vi "Bring To Cursor.vi"(8 "error in (no error)":errorcluster, 11 "Palette Data":T1) -> (0 "error out":errorcluster)   [LabVIEW 2014, in "SmartPalette.lvlib"]
uses:
  SmartPalette.lvlib
  Controls/Palette Data.ctl
  <vilib>/picture/picture.llb/imagedata.ctl
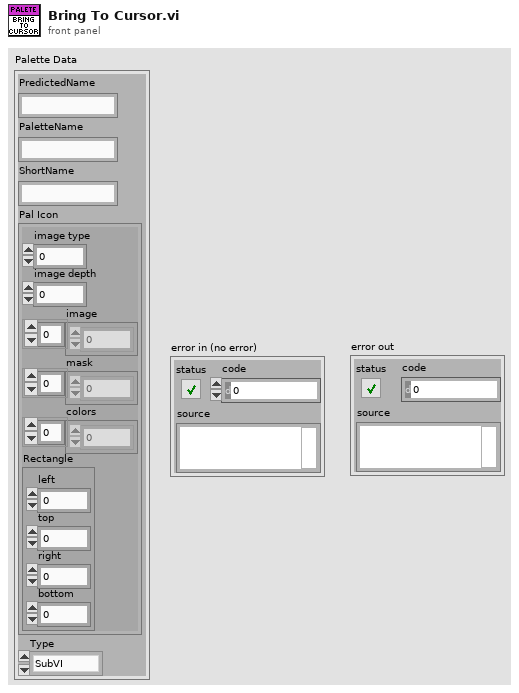
[diagram p1: front panel]
types:
  T1 = typedef "SmartPalette.lvlib/Palette Data.ctl" = cluster{"PredictedName":string, "PaletteName":string, "ShortName":string, "Pal Icon":T2, "Type":enum16{"SubVI", "VI Templtate", "Function"}}
  T2 = typedef "imagedata.ctl" = cluster{"image type":i32, "image depth":i32, "image":u8[], "mask":u8[], "colors":u32[], "Rectangle":cluster{"left":i16, "top":i16, "right":i16, "bottom":i16}}
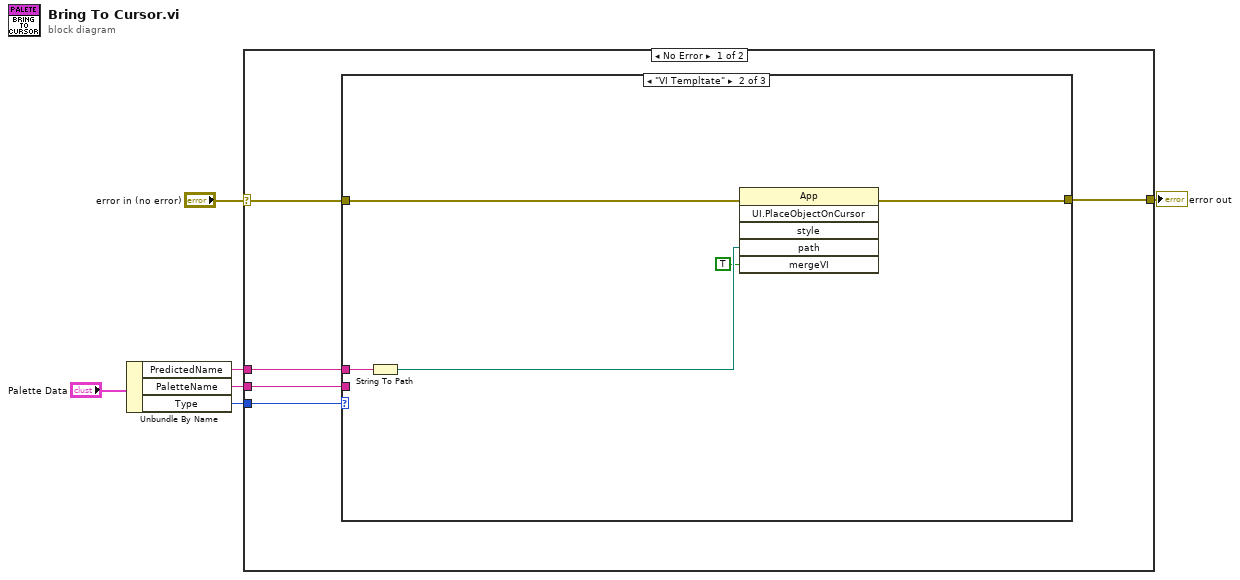
[diagram p0: block diagram]
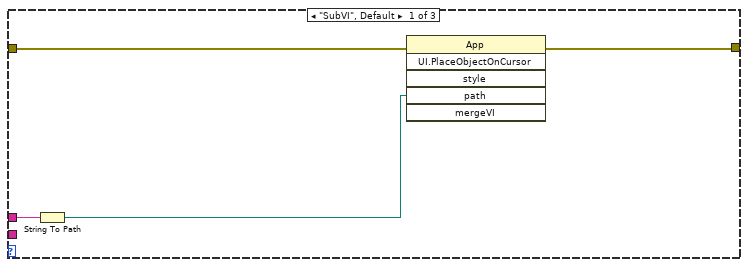
[diagram p2: hidden frame]
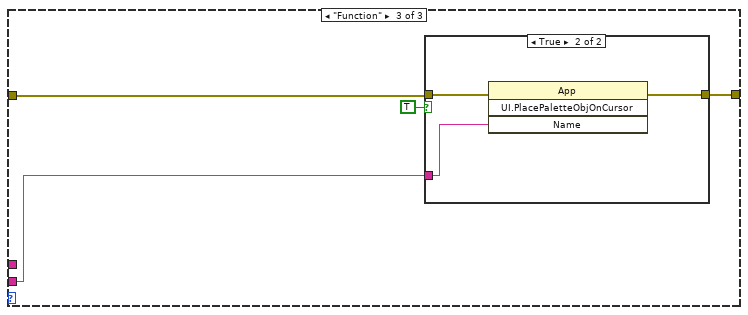
[diagram p3: hidden frame]
diagram:
  n1 = Unbundle By Name("Palette Data") -> ("PredictedName"=w1:string, "PaletteName"=w2:string, "Type"=w3:enum16{"SubVI", "VI Templtate", "Function"})
  n2 = case shown="No Error" "error in (no error)" {
    selector: "error in (no error)" -> [w10 w28]
    tunnel: [w11 w28] -> w6
    tunnel: w3 -> [w9 _]
    tunnel: w2 -> [w8 _]
    tunnel: w1 -> [w7 _]
    frame No Error {
      n3 = case shown="\"VI Templtate\"" w9 {
        tunnel: [w13 w18 w24] -> w11
        tunnel: w10 -> [w14 w19 w21]
        tunnel: w8 -> [_ _ w22]
        tunnel: w7 -> [w15 w20 _]
        frame "SubVI", Default {
          n4 = String To Path(string=w15) -> (path=w12:path)
          n5 = invoke class="App" method="UI.PlaceObjectOnCursor"(error in=w14, "path"=w12) -> (error out=w13:errorcluster)  [unwired: 4 in, 5 out]
        }
        frame "VI Templtate" {
          n6 = String To Path(string=w20) -> (path=w17:path)
          n7 = invoke class="App" method="UI.PlaceObjectOnCursor"(error in=w19, "path"=w17, "mergeVI"=TRUE) -> (error out=w18:errorcluster)  [unwired: 3 in, 5 out]
        }
        frame "Function" {
          n8 = case shown="True" TRUE {
            tunnel: [_ w27] -> w24
            tunnel: w22 -> [_ w26]
            tunnel: w21 -> [_ w25]
            frame False {
            }
            frame True {
              n9 = invoke class="App" method="UI.PlacePaletteObjOnCursor"(error in=w25, "Name"=w26) -> (error out=w27:errorcluster)  [unwired: 2 in, 3 out]
            }
          }
        }
      }
    }
    frame Error {
    }
  }
  "error out" <- w6
